vi "QSM_Push to Queue.vi"(6 "Push to FRONT of Queue?":bool, 8 "error in (no error)":errorcluster, 9 "Data (Variant)":variant, 10 "QSM_RunStates_TEST":T2, 11 "QSM_Reference_TEST":T1) -> (0 "error out":errorcluster, 3 "QSM_Reference_TESTOut":T1)   [LabVIEW 2014, in "TestQSM.lvlib"]
uses:
  TestQSM.lvlib
  Controls/QSM_RunStates.ctl
  Controls/QSM_Reference.ctl
  Controls/QSM_DataType.ctl
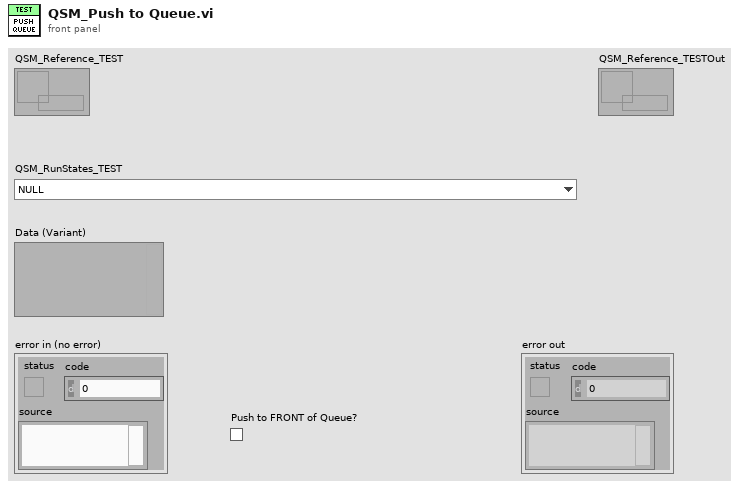
[diagram p1: front panel]
types:
  T1 = typedef "TestQSM.lvlib/QSM_Reference.ctl" = refnum<queue>
  T2 = typedef "TestQSM.lvlib/QSM_RunStates.ctl" = enum16{"NULL", "Sect01-Initialize-00-GROUP.ENQUEUE", "Sect02-Single File_Check for Parameters", "Sect02-Single File_Ask for File", "Sect02-Single File_Run Analysis", "Sect02-Single File_Write Results", "Sect03-Single ROI Calc_Check for Parameters", "Sect03-Single ROI Calc_Ask for File", "Sect03-Single ROI Calc_Run Analysis", "Sect03-Single ROI _Write Results", "Sect12-Full Dir_Check for Parameters", "Sect12-Full Dir_Ask for Dir", "Sect12-Full Dir_Check for Next Image to Process", "Sect12-Full Dir_Run Analysis", "Sect12-Full Dir_Write Results", "Sect12-Full Dir_Check if User Stopped", "Sect13-FullDir ROI Calc_Check for Parameters", "Sect13-FullDir ROI Calc_Ask for Dir", "Sect13-Full Dir ROI Calc_Check for Next Image to Process", "Sect13-Full Dir ROI Calc_Run Analysis", "Sect13-Full Dir ROI Calc_Write Results", "Sect13-Full Dir ROI Calc_Check if User Stopped", "Sect90-GUI_Config_Change UI Before Analysis", "Sect90-GUI_Config_Change UI After Analysis", "Sect90-GUI_Stop Processing Pressed", "Sect90-GUI_Stop Processing Button Set Back to F", "Sect90-GUI_Clear ROIs", "Sect99_EXIT-00-Group.Enqueue", "Sect99_EXIT-01-StopQSM"}
  T3 = typedef "TestQSM.lvlib/QSM_DataType.ctl" = cluster{"RunStates":T2, "Data (Variant)":variant}
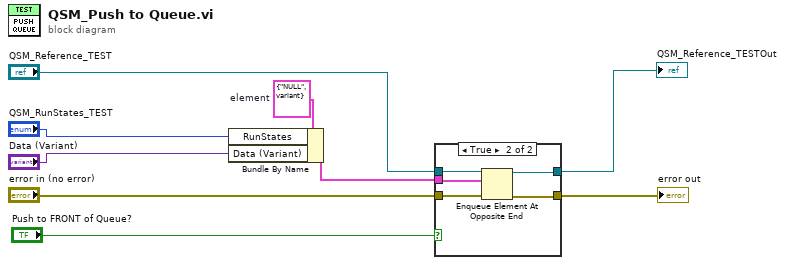
[diagram p0: block diagram]
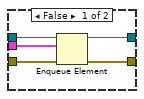
[diagram p2: hidden frame]
diagram:
  w7 = T3 {"RunStates"=enum."NULL", "Data (Variant)"=variant}  # element
  n1 = Bundle By Name(cluster=w7, "RunStates"="QSM_RunStates_TEST", "Data (Variant)"="Data (Variant)") -> (w3:T3)
  n2 = case shown="True" "Push to FRONT of Queue?" {
    tunnel: w3 -> [w14 w16]
    tunnel: [w13 w15] -> w1
    tunnel: "error in (no error)" -> [w12 w17]
    tunnel: "QSM_Reference_TEST" -> [w11 w19]
    tunnel: [w10 w18] -> w2
    frame False {
      n3 = Enqueue Element(queue=w11, element=w14, error in (no error)=w12) -> (queue out=w10:T1, error out=w13:errorcluster)  [unwired: 1 in, 1 out]
    }
    frame True {
      n4 = Enqueue Element At Opposite End(queue=w19, element=w16, error in (no error)=w17) -> (queue out=w18:T1, error out=w15:errorcluster)  [unwired: 1 in, 1 out]
    }
  }
  "error out" <- w1
  "QSM_Reference_TESTOut" <- w2
